vi "new Room.vi"(8 "error in (no error)":errorcluster, 10 "roomNumber":i32) -> (0 "error out":errorcluster, 3 "Room* out":refnum<data-value>)   [LabVIEW 2016, in "Room.lvclass"]
uses:
  Room.lvclass
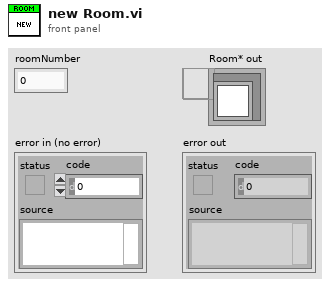
[diagram p1: front panel]
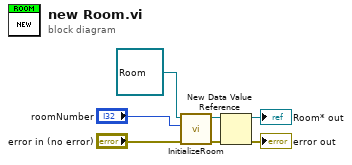
[diagram p0: block diagram]
diagram:
  n1 = call "InitializeRoom.vi"("error in (no error)"="error in (no error)", "roomNumber"="roomNumber", "Room in"=refnum<class "Room.lvclass"> refnum) -> ("error out"=w1:errorcluster, "Room out"=w5:refnum<class "Room.lvclass">)  [unwired: 7 in]
  n2 = New Data Value Reference(data value=w5, error in=w1) -> (data value reference=→"Room* out":refnum<data-value>, error out=→"error out":errorcluster)
